vi "Update Analog Config.vi"(8 "error in (no error)":errorcluster, 11 "Señal Analogica":T1={"Canal/Canales"="", "Canal"="DAQSim1", "Canales"=[], "Frecuencia de muestreo"=1000, "Numero de muestras"=1000, "Tiempo de AQ"=0.0}) -> (0 "error out":errorcluster)   [LabVIEW 2020, in "Settings.lvlib"]
uses:
  Settings.lvlib
  Aqcisition/Analog Signal Config.ctl
  <vilib>/drjdpowell/SQLite Library/SQL Connection/Open (path).vi
  <vilib>/drjdpowell/SQLite Library/SQL Connection/Open (string).vi
  <vilib>/AdvancedString/Path To Command Line String.vi
  <vilib>/drjdpowell/SQLite Library/SQL Connection/Execute SQL (No results).vi
  <vilib>/drjdpowell/SQLite Library/SQL Connection/Connection.lvclass
  <vilib>/drjdpowell/SQLite Library/SQLite.lvlib
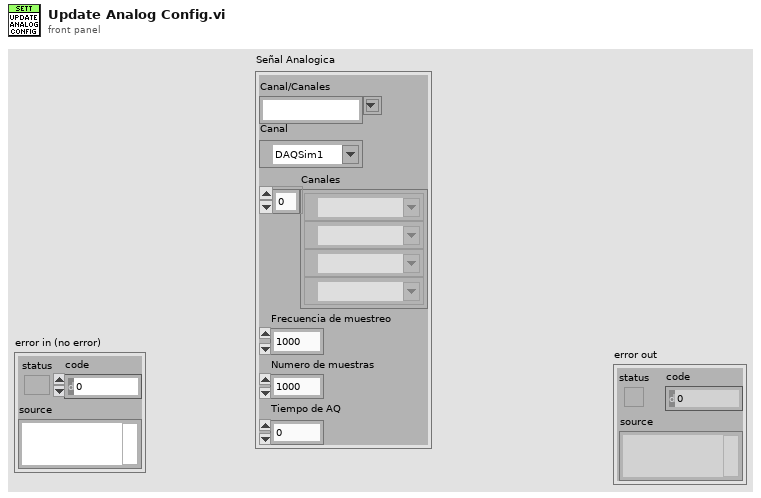
[diagram p1: front panel]
types:
  T1 = typedef "Analog Signal Config.ctl" = cluster{"Canal/Canales":string, "Canal":tag, "Canales":tag[], "Frecuencia de muestreo":i32, "Numero de muestras":i32, "Tiempo de AQ":dbl}
  T2 = cluster{"Canales[0]":tag, "Canales[1]":tag, "Canales[2]":tag, "Canales[3]":tag, "Canales[4]":tag, "Canales[5]":tag, "Canales[6]":tag, "Canales[7]":tag, "Canales[8]":tag}
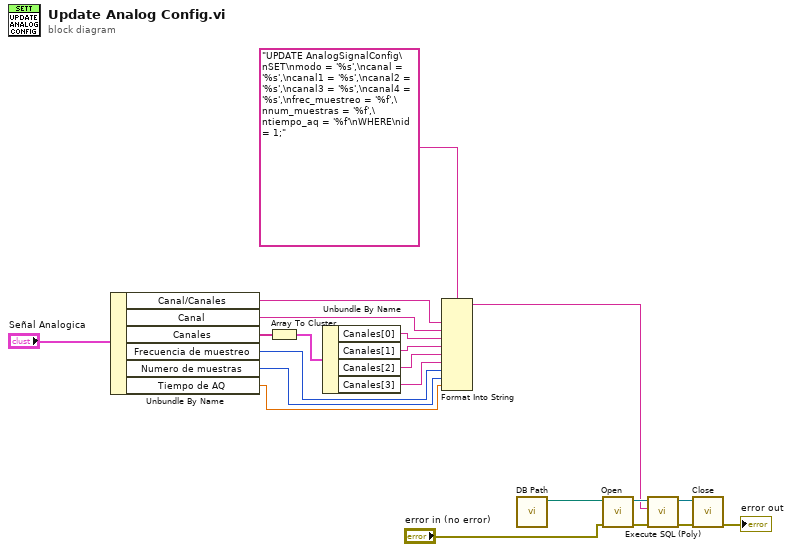
[diagram p0: block diagram]
diagram:
  n1 = Unbundle By Name("Señal Analogica") -> ("Canal/Canales"=w13:string, "Canal"=w12:tag, "Canales"=w9:tag[], "Frecuencia de muestreo"=w3:i32, "Numero de muestras"=w2:i32, "Tiempo de AQ"=w1:dbl)
  n2 = Array To Cluster(array=w9) -> (cluster=w8:T2)
  n3 = Unbundle By Name(w8) -> ("Canales[0]"=w7:tag, "Canales[1]"=w6:tag, "Canales[2]"=w5:tag, "Canales[3]"=w4:tag)
  n4 = Format Into String(format string="UPDATE AnalogSignalConfig\nSET\nmodo = '%s',\ncanal = '%s',\ncanal1 = '%s',\ncanal2 = '%s',\ncanal3 = '%s',\ncanal4 = '%s',\nfrec_muestreo = '%f',\nnum_muestras = '%f',\ntiempo_aq = '%f'\nWHERE\nid = 1;", w13, w12, w7, w6, w5, w4, w3, w2, w1) -> (resulting string=w11:string)  [unwired: 2 in, 1 out]
  n5 = call "DB Path.vi"() -> ("appended path"=w14:path)  [unwired: 11 in]
  n6 = call-poly <vilib>:"Open.vi"("error in (no error)"="error in (no error)", "db file"=w14) -> ("error out"=w21:errorcluster, "SQLite Connection"=w20:refnum<class "Connection.lvclass">)  [unwired: 8 in]
  n7 = call-poly <vilib>:"Execute SQL (Poly).vi"("error in (no error)"=w21, "SQL"=w11, "SQLite Connection in"=w20) -> ("error out"=w19:errorcluster, "SQLite Connection"=w18:refnum<class "Connection.lvclass">)  [unwired: 7 in]
  n8 = call-dynamic "Close.vi"("error in (no error)"=w19, "SQLite Connection in"=w18) -> ("error out"=→"error out":errorcluster)  [unwired: 9 in]
